vi "AllRefDelete.vi"(8 "error in (no error)":errorcluster caption="错误输入（无错误）", 11 "MainPage 输入":refnum<class "MainPage.lvclass">) -> (0 "error out":errorcluster caption="错误输出", 3 "MainPage 输出":refnum<class "MainPage.lvclass">)   [LabVIEW 2019, in "MainPage.lvlib" / "MainPage.lvclass"]
uses:
  MainPage.lvclass
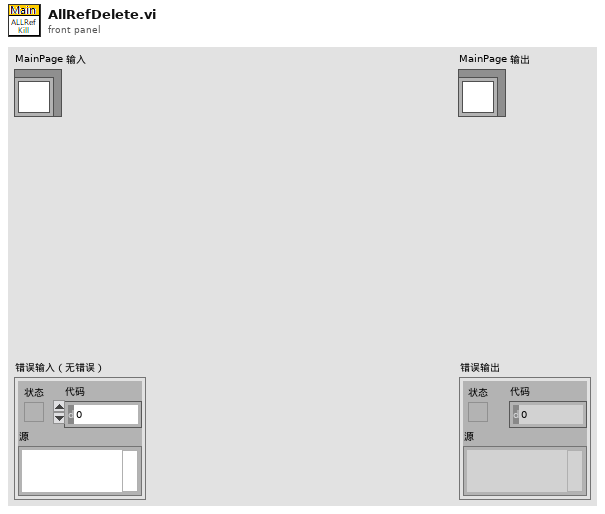
[diagram p1: front panel]
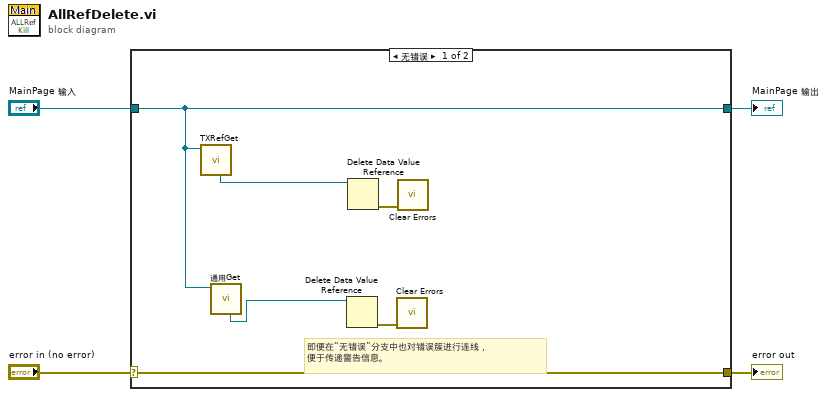
[diagram p0: block diagram]
diagram:
  n1 = case shown="无错误" "error in (no error)" {
    selector: "error in (no error)" -> [w10 w12]
    tunnel: [w10 w12] -> w3
    tunnel: [w7 w11] -> w1
    tunnel: "MainPage 输入" -> [w7 w11]
    frame No Error {
      # "即便在“无错误”分支中也对错误簇进行连线，\n便于传递警告信息。"
      n2 = call-dynamic "TXRefGet.vi"("MainPage 输入"=w7) -> ("引用"=w8:refnum<data-value>)  [unwired: 6 in, 4 out]
      n3 = call-dynamic "通用Get.vi"("MainPage 输入"=w7) -> ("通用引用"=w5:refnum<data-value>)  [unwired: 6 in, 4 out]
      n4 = Delete Data Value Reference(data value reference=w5) -> (error out=w6:errorcluster)  [unwired: 1 in, 1 out]
      n5 = Delete Data Value Reference(data value reference=w8) -> (error out=w9:errorcluster)  [unwired: 1 in, 1 out]
      n6 = call <vilib>:"Clear Errors.vi"("error in (no error)"=w6) -> ()  [unwired: 5 in, 2 out]
      n7 = call <vilib>:"Clear Errors.vi"("error in (no error)"=w9) -> ()  [unwired: 5 in, 2 out]
    }
    frame Error {
    }
  }
  "error out" <- w3
  "MainPage 输出" <- w1
